vi "Get Base Protocol.vi"(8 "error in (no error)":errorcluster, 11 "RS232 in":refnum<class "RS-xxx.lvclass">) -> (0 "error out":errorcluster, 2 "Protocol out":T1, 3 "RS232 out":refnum<class "RS-xxx.lvclass">)   [LabVIEW 2019, in "Localhost Protocols.lvlib" / "RS-xxx.lvclass"]
uses:
  RS-xxx.lvclass
  Protocol Parent/Types/Base Protocol Type.ctl
  Protocol Parent/Protocol Parent.lvclass
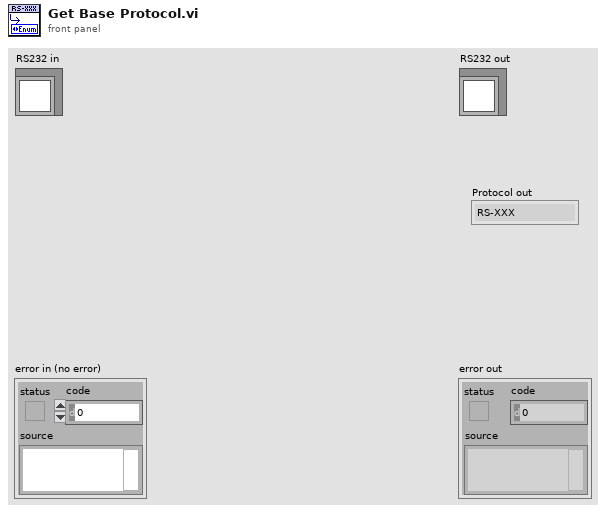
[diagram p1: front panel]
types:
  T1 = typedef "Localhost Protocols.lvlib/Protocol Parent.lvclass/Base Protocol Type.ctl" = enum16{"RS-XXX", "VISA", "TCPIP", "UDP", "GPIB ConvBox"}
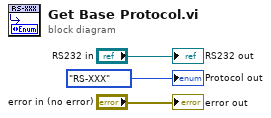
[diagram p0: block diagram]
diagram:
  "error out" <- "error in (no error)"
  "RS232 out" <- "RS232 in"
  "Protocol out" <- Base_Protocol_Type."RS-XXX" ("Protocol out")
